vi "H Drive.vi"(0 "Y Power":dbl, 1 "Strafe Correct Tolerance":dbl, 2 "Strafe Correct PID Gains":T1={"proportional gain (Kc)"=1.0, "integral time (Ti, min)"=0.01, "derivative time (Td, min)"=0.0} {"derivative time (Td, min)" format="%.3f"; "integral time (Ti, min)" format="%.3f"; "proportional gain (Kc)" format="%.3f"}, 5 "Turn Power":dbl, 7 "Strafe Power":dbl, 9 "Center Piston Down?":bool, 11 "Traction?":bool, 12 "Strafe Correct":bool) -> (4 "X Out":dbl, 6 "Y out":dbl, 8 "Center Motor Output":dbl, 10 "HDrive Piston":bool, 15 "Grasshopper Pistons":bool)   [LabVIEW 2016]
uses:
  Common Code/PID Gains.ctl
  Common Code/Utilities/Change Detect Boolean.vi
  Common Code/Utilities/Change Detect Double.vi
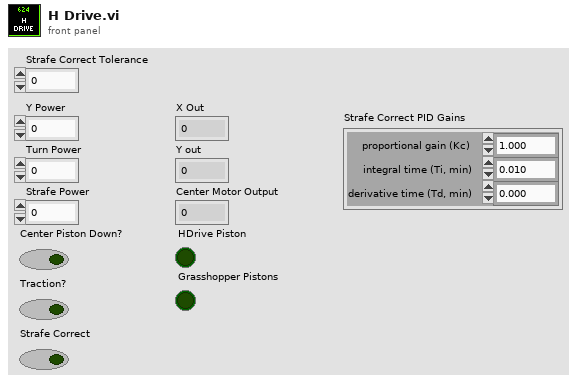
[diagram p1: front panel]
types:
  T1 = typedef "PID Gains.ctl" = cluster{"proportional gain (Kc)":dbl, "integral time (Ti, min)":dbl, "derivative time (Td, min)":dbl}
  T2 = cluster{"Yaw":dbl, "Roll":dbl, "Pitch":dbl, "Heading":dbl, "Fused Heading":dbl}
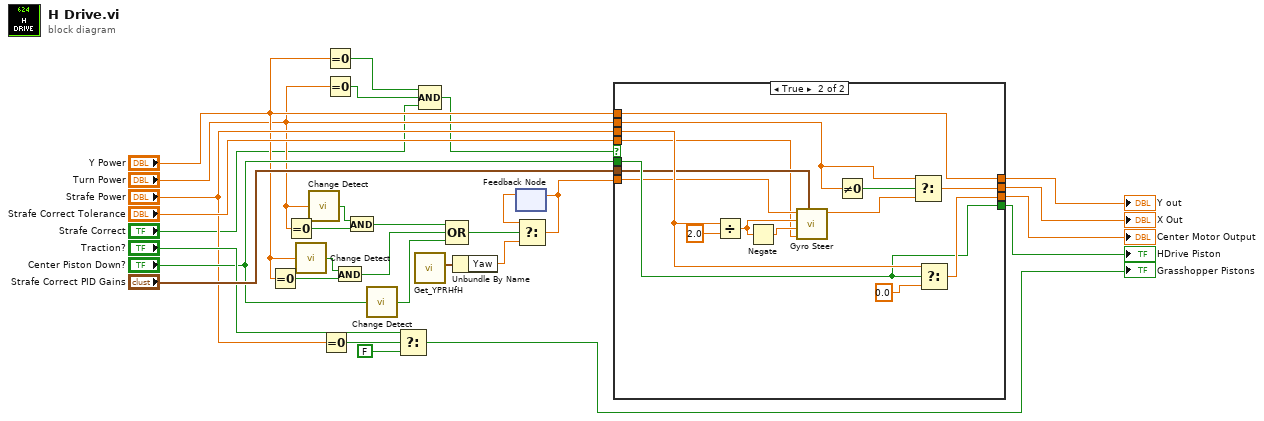
[diagram p0: block diagram]
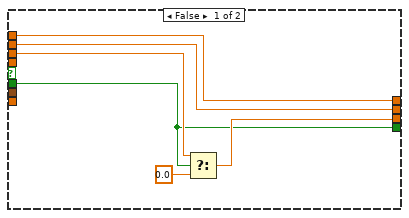
[diagram p2: hidden frame]
diagram:
  n1 = Equal To 0?(x="Y Power") -> (x = 0?=w18:bool)
  n2 = Equal To 0?(x="Turn Power") -> (x = 0?=w11:bool)
  n3 = call-poly "Change Detect.vi"("In"="Y Power") -> ("Changed?"=w17:bool)
  n4 = call-poly "Change Detect.vi"("In"="Turn Power") -> ("Changed?"=w12:bool)
  n5 = Equal To 0?(x="Strafe Power") -> (x = 0?=w26:bool)
  n6 = Equal To 0?(x="Y Power") -> (x = 0?=w4:bool)
  n7 = Equal To 0?(x="Turn Power") -> (x = 0?=w3:bool)
  n8 = And(x=w17, y=w18) -> (x .and. y?=w13:bool)
  n9 = And(x=w12, y=w11) -> (x .and. y?=w10:bool)
  n10 = call-poly "Change Detect.vi"("In"="Center Piston Down?") -> ("Changed?"=w15:bool)
  n11 = Select(t="Traction?", s=w26, f=FALSE ("t")) -> (s? t:f=→"Grasshopper Pistons":bool)
  n12 = call <vilib>:"Get_YPRHfH.vi"() -> ("YRPHfH"=w22:T2)  [unwired: 11 in]
  n13 = Compound Arithmetic op=AND(w4, w3, "Strafe Correct") -> (w1:bool)
  n14 = Compound Arithmetic op=OR(w10, w13, w15) -> (w14:bool)
  n15 = Unbundle By Name(w22) -> ("Yaw"=w19:dbl)
  n16 = feedback #1() -> (w21:dbl)  [unwired: 1 in]
  n17 = Select(t=w21, s=w14, f=w19) -> (s? t:f=w20:dbl)
  n18 = feedback-in #1(w20) -> ()
  n19 = case shown="True" w1 {
    tunnel: "Strafe Power" -> [w35 w44]
    tunnel: "Center Piston Down?" -> [w31 w42]
    tunnel: [w34 w43] -> w7
    tunnel: [w31 w42] -> w30
    tunnel: "Strafe Correct PID Gains" -> [_ w41]
    tunnel: "Y Power" -> [w33 w46]
    tunnel: [w33 w46] -> w28
    tunnel: "Turn Power" -> [w32 w47]
    tunnel: [w32 w49] -> w27
    tunnel: w20 -> [_ w40]
    tunnel: "Strafe Correct Tolerance" -> [_ w37]
    frame False {
      n20 = Select(t=w35, s=w31, f=0.0) -> (s? t:f=w34:dbl)
    }
    frame True {
      n21 = Divide(x=w44, y=2.0) -> (x/y=w39:dbl)
      n22 = Negate(x=w39) -> (-x=w38:dbl)
      n23 = call "Gyro Steer.vi"("PID gains"=w41, "Gyro Tolerance"=w37, "X Min Output"=w38, "X Max Output"=w39, "Target Heading"=w40) -> ("X out"=w48:dbl)  [unwired: 5 in, 1 out]
      n24 = Not Equal To 0?(x=w47) -> (x != 0?=w50:bool)
      n25 = Select(t=w47, s=w50, f=w48) -> (s? t:f=w49:dbl)
      n26 = Select(t=w44, s=w42, f=0.0) -> (s? t:f=w43:dbl)
    }
  }
  "Center Motor Output" <- w7
  "HDrive Piston" <- w30
  "X Out" <- w27
  "Y out" <- w28
